vi "Draw Legend.vi"(7 "Mode":enum16{"Horizontal", "Vertical"}(ring), 8 "error in (no error)":errorcluster caption="错误输入（无错误）", 9 "Legend Info":T1={"Name"="", "Percent"=0.0, "TxtColor"=0, "Hor Space"=5, "Ver Space"=5, "Color Segement"=[16448250, 0, 16736786, 1198079]}, 10 "origin":cluster{"x":i16, "y":i16} caption="Origin", 11 "Gradient PieChart 输入":refnum<class "Gradient PieChart.lvclass"> caption="DNL_LabVIEW Object in") -> (0 "error out":errorcluster caption="错误输出", 2 "Next Origin":cluster{"x":i16, "y":i16} caption="Next Orgin", 3 "Gradient PieChart 输出":refnum<class "Gradient PieChart.lvclass"> caption="DNL_LabVIEW Object out")   [LabVIEW 2012, in "Picture Box Tools.lvlib" / "Gradient PieChart.lvclass"]
uses:
  Gradient PieChart.lvclass
  Legend Info.ctl
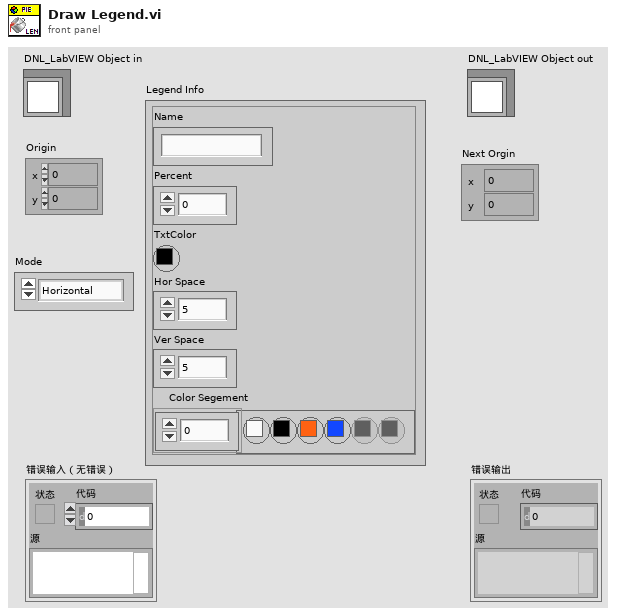
[diagram p1: front panel]
types:
  T1 = typedef "Picture Box Tools.lvlib/Gradient PieChart.lvclass/Legend Info.ctl" = cluster{"Name":string, "Percent":dbl, "TxtColor":u32, "Hor Space":i16, "Ver Space":i16, "Color Segement":u32[]}
  T2 = cluster{"left":i16, "top":i16, "right":i16, "bottom":i16}
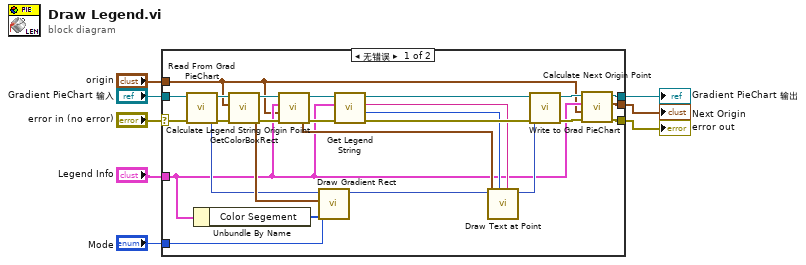
[diagram p0: block diagram]
diagram:
  n1 = case shown="无错误" "error in (no error)" {
    selector: "error in (no error)" -> [w33 w36]
    tunnel: [w12 w36] -> w7
    tunnel: [w13 w35] -> w5
    tunnel: "Gradient PieChart 输入" -> [w30 w35]
    tunnel: "origin" -> [w9 _]
    tunnel: "Legend Info" -> [w10 _]
    tunnel: "Mode" -> [w26 _]
    tunnel: [w11 _] -> w1
    frame No Error {
      n2 = call "Read From Grad PieChart.vi"("error in (no error)"=w33, "Gradient PieChart输入"=w30) -> ("error out"=w31:errorcluster, "Grad PieChart"=w28:picture, "Gradient PieChart输出"=w32:refnum<class "Gradient PieChart.lvclass">)  [unwired: 7 in]
      n3 = Unbundle By Name(w10) -> ("Color Segement"=w27:u32[])
      n4 = call "GetColorBoxRect.vi"("error in (no error)"=w31, "origin"=w9, "Gradient PieChart 输入"=w32) -> ("error out"=w24:errorcluster, "ColorBoxRect"=w29:T2, "Gradient PieChart 输出"=w23:refnum<class "Gradient PieChart.lvclass">)  [unwired: 6 in]
      n5 = call "Calculate Legend String Origin Point.vi"("error in (no error)"=w24, "origin"=w9, "Legend Info"=w10, "Gradient PieChart 输入"=w23) -> ("error out"=w20:errorcluster, "Next Origin"=w22:cluster{"x":i16, "y":i16}, "Gradient PieChart 输出"=w21:refnum<class "Gradient PieChart.lvclass">)  [unwired: 5 in]
      n6 = call "Draw Gradient Rect.vi"("Color Segement"=w27, "Mode"=w26, "rect"=w29, "picture in"=w28) -> ("picture out"=w25:picture)  [unwired: 7 in]
      n7 = call "Get Legend String.vi"("error in (no error)"=w20, "Legend Info"=w10, "Gradient PieChart 输入"=w21) -> ("error out"=w18:errorcluster, "TxtColor"=w16:u32, "Legend String"=w17:string, "Gradient PieChart 输出"=w19:refnum<class "Gradient PieChart.lvclass">)  [unwired: 5 in]
      n8 = call <vilib>:"Draw Text at Point.vi"("text color(black)"=w16, "text"=w17, "origin"=w22, "picture"=w25) -> ("new picture"=w34:picture)  [unwired: 6 in, 1 out]
      n9 = call "Write to Grad PieChart.vi"("error in (no error)"=w18, "Grad PieChart"=w34, "Gradient PieChart输入"=w19) -> ("error out"=w14:errorcluster, "Gradient PieChart输出"=w15:refnum<class "Gradient PieChart.lvclass">)  [unwired: 7 in]
      n10 = call "Calculate Next Origin Point.vi"("error in (no error)"=w14, "origin"=w9, "Legend Info"=w10, "Gradient PieChart 输入"=w15) -> ("error out"=w12:errorcluster, "Next Origin"=w11:cluster{"x":i16, "y":i16}, "Gradient PieChart 输出"=w13:refnum<class "Gradient PieChart.lvclass">)  [unwired: 5 in]
    }
    frame Error {
    }
  }
  "error out" <- w7
  "Gradient PieChart 输出" <- w5
  "Next Origin" <- w1
